vi "Get stack name.vi"(0 "Module?":bool, 1 "Baseplate Type":string, 5 "Protoname (baselayer)":string="320-PH-F2CX-CM-0055", 7 "Sensor thickness":string, 9 "Geometry":string="XX-", 11 "Resolution":string="HD", 14 "Hexaboard ROC version":string="X") -> (8 "Stack name":string="320-PH-F1-CM-0054")   [LabVIEW 2021, in "Stack.lvclass"]
uses:
  Stack.lvclass
  <vilib>/JDP Science/JDP Science Common Utilities/JDP Utility.lvlib
panel:
  out "Institution":string="CM"
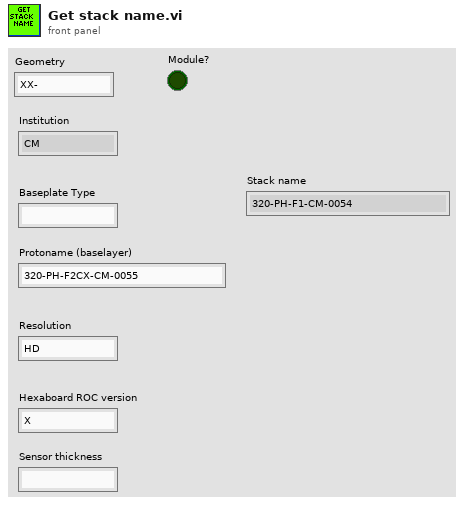
[diagram p1: front panel]
types:
  T1 = typedef "File Paths.ctl" = cluster{"Glue Pattern Folder":path, "Carrier Tray Folder":path, "Pick Up Tool Fixture Folder":path, "Components Folder":path, "Bellows Tool Offset.txt":path, "Pick Up Tool Offset.txt":path, "Dispense Tip Offset.txt":path, "Log Files":path, "Gantry Assembly Map.txt":path, "Syringe and offset map.txt":path, "Controllers Folder":path, "Local dbase config":path}
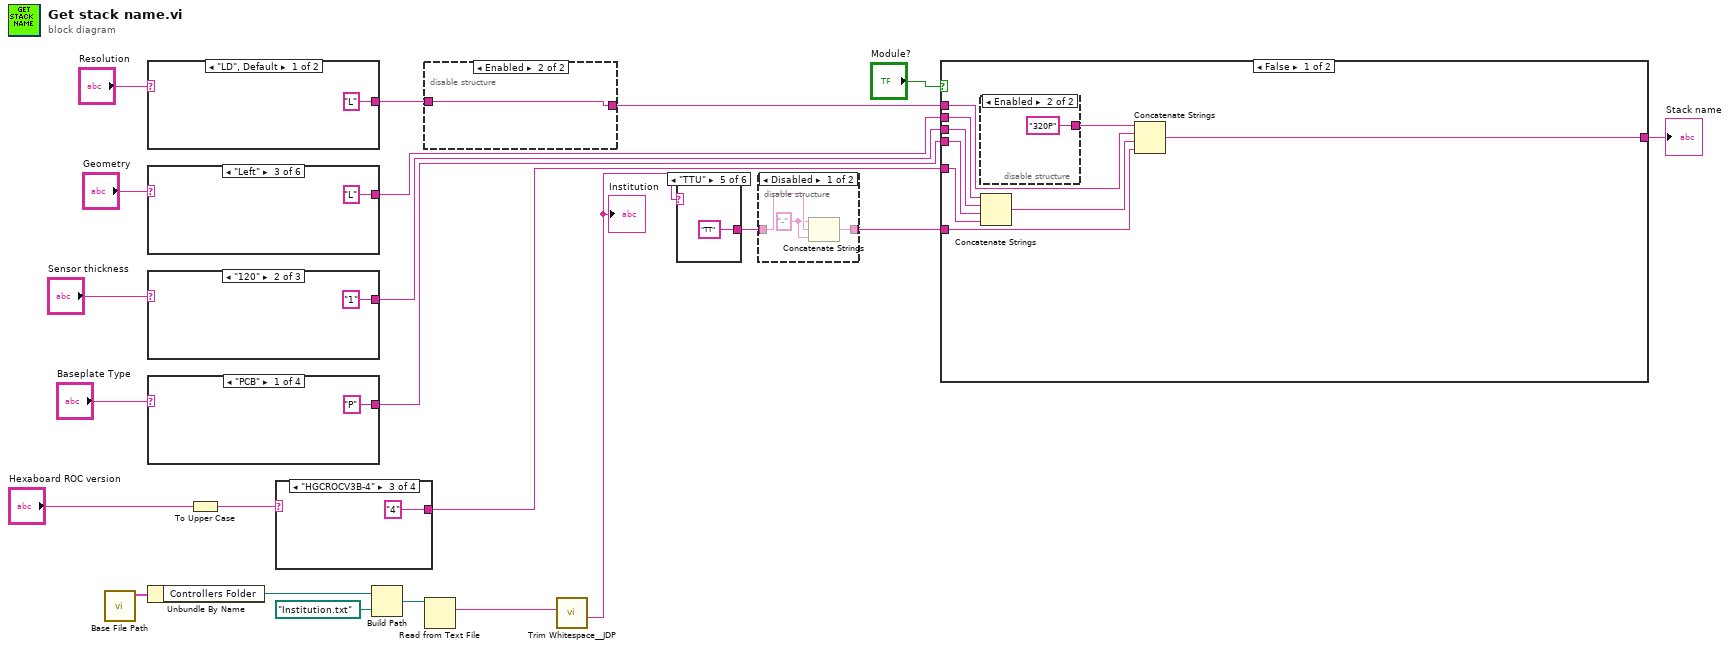
[diagram p0: block diagram]
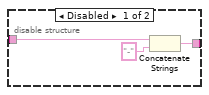
[diagram p2: hidden frame]
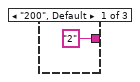
[diagram p4: hidden frame]
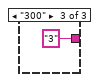
[diagram p5: hidden frame]
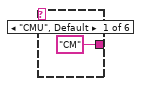
[diagram p6: hidden frame]
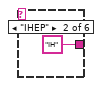
[diagram p7: hidden frame]
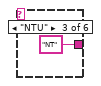
[diagram p8: hidden frame]
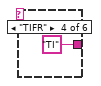
[diagram p9: hidden frame]
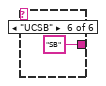
[diagram p10: hidden frame]
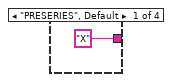
[diagram p11: hidden frame]
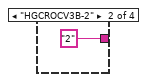
[diagram p12: hidden frame]
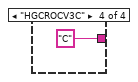
[diagram p13: hidden frame]
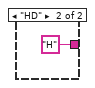
[diagram p14: hidden frame]
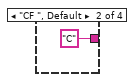
[diagram p15: hidden frame]
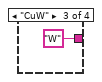
[diagram p16: hidden frame]
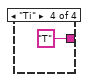
[diagram p17: hidden frame]
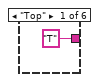
[diagram p18: hidden frame]
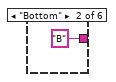
[diagram p19: hidden frame]
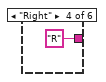
[diagram p20: hidden frame]
diagram:
  n1 = call "Base File Path.vi"() -> ("Paths Out"=w12:T1)  [unwired: 11 in]
  n2 = case shown="\"LD\", Default" "Resolution" {
    tunnel: ["L" "H"] -> w2
    frame "LD", Default {
    }
    frame "HD" {
    }
  }
  n3 = case shown="\"Left\"" "Geometry" {
    tunnel: ["T" "B" "L" "R" "5" "F"] -> w18
    frame "Top" {
    }
    frame "Bottom" {
    }
    frame "Left" {
    }
    frame "Right" {
    }
    frame "Five" {
    }
    frame "Full", Default {
    }
  }
  n4 = case shown="\"120\"" "Sensor thickness" {
    tunnel: ["2" "1" "3"] -> w5
    frame "200", Default {
    }
    frame "120" {
    }
    frame "300" {
    }
  }
  n5 = case shown="\"PCB\"" "Baseplate Type" {
    tunnel: ["P" "C" "W" "T"] -> w15
    frame "PCB" {
    }
    frame "CF ", Default {
    }
    frame "CuW" {
    }
    frame "Ti" {
    }
  }
  n6 = Unbundle By Name(w12) -> ("Controllers Folder"=w11:path)
  n7 = To Upper Case(1:"Hexaboard ROC version") -> (0:w3:string)
  n8 = case shown="\"HGCROCV3B-4\"" w3 {
    tunnel: ["X" "2" "4" "C"] -> w14
    frame "PRESERIES", Default {
    }
    frame "HGCROCV3B-2" {
    }
    frame "HGCROCV3B-4" {
    }
    frame "HGCROCV3C" {
    }
  }
  n9 = Build Path(base path=w11, name or relative path=path "Institution.txt") -> (appended path=w9:path)
  n10 = disable-structure shown="Enabled" {
    disable-tunnel: w2 -> [w44 w45]
    disable-tunnel: [w42 w45] -> w1
    frame Disabled {
      n11 = Concatenate Strings(w44, "-" ("string")) -> (w42:string)
    }
    frame Enabled {
    }
  }
  n12 = Read from Text File(file (use dialog)=w9) -> (text=w8:string)  [unwired: 3 in, 3 out]
  n13 = call <vilib>:"Trim Whitespace__JDP.vi"("String in"=w8) -> ("String out"=w7:string)  [unwired: 6 in]
  "Institution" <- w7
  n14 = case shown="\"TTU\"" w7 {
    tunnel: ["CM" "IH" "NT" "TI" "TT" "SB"] -> w13
    frame "CMU", Default {
    }
    frame "IHEP" {
    }
    frame "NTU" {
    }
    frame "TIFR" {
    }
    frame "TTU" {
    }
    frame "UCSB" {
    }
  }
  n15 = disable-structure shown="Disabled" {
    disable-tunnel: [w54 w55] -> w21
    disable-tunnel: w13 -> [w53 w55]
    frame Disabled {
      w52 = "-" ("string")
      n16 = Concatenate Strings(w52, w53, w52) -> (w54:string)
    }
    frame Enabled {
    }
  }
  n17 = case shown="False" "Module?" {
    tunnel: [w58 w69] -> w20
    tunnel: w21 -> [w63 _]
    tunnel: w18 -> [w62 _]
    tunnel: w1 -> [w56 _]
    tunnel: w5 -> [w64 _]
    tunnel: w15 -> [w60 _]
    tunnel: w14 -> [w59 _]
    frame False {
      n18 = disable-structure shown="Enabled" {
        disable-tunnel: ["320-P" ("string") "320P" ("string")] -> w57
        frame Disabled {
        }
        frame Enabled {
        }
      }
      n19 = Concatenate Strings(w62, w64, w60, w59) -> (w61:string)
      n20 = Concatenate Strings(w57, w56, w61, w63) -> (w58:string)
    }
    frame True {
      n21 = To Upper Case(1:"Protoname (baselayer)") -> (0:w67:string)
      n22 = Search and Replace String(replace all?=TRUE ("replace all? (F)"), input string=w67, search string="-") -> (result string=w71:string)  [unwired: 5 in, 3 out]
      n23 = String Subset(string=w71, length (rest)=1 ("length (rest)")) -> (substring=w72:string)  [unwired: 1 in]
      n24 = case shown="\"P \", Default" w72 {
        tunnel: w71 -> [w95 w98]
        tunnel: [w93 w97] -> w70
        frame "P ", Default {
          n25 = String Subset(string=w95, offset (0)=1 ("length (rest)")) -> (substring=w93:string)  [unwired: 1 in]
        }
        frame "3" {
          n26 = String Subset(string=w98, offset (0)=4) -> (substring=w97:string)  [unwired: 1 in]
        }
      }
      n27 = disable-structure shown="Enabled" {
        disable-tunnel: w70 -> [w88 w90]
        disable-tunnel: [w76 w91] -> w69
        frame Disabled {
          w83 = "-" ("string")
          n28 = String Subset(string=w88, length (rest)=1 ("length (rest)")) -> (substring=w87:string)  [unwired: 1 in]
          n29 = String Subset(string=w88, offset (0)=1, length (rest)=4 ("length (rest)")) -> (substring=w86:string)
          n30 = String Subset(string=w88, offset (0)=5, length (rest)=2 ("length (rest)")) -> (substring=w85:string)
          n31 = String Subset(string=w88, offset (0)=7) -> (substring=w84:string)  [unwired: 1 in]
          n32 = Concatenate Strings("320-M" ("string"), w87, w83, w86, w83, w85, w83, w84) -> (w76:string)
        }
        frame Enabled {
          n33 = Concatenate Strings("320M" ("string"), w90) -> (w91:string)
        }
      }
    }
  }
  "Stack name" <- w20
